vi "AMSServer.vi"() -> ()   [LabVIEW 2013]
uses:
  Controls/Enum - AMSServer State.ctl
  Controls/General Settings - AMS.ctl
  Controls/Configure Parameters - AMS.ctl
  Controls/Simulate Parameters - AMS.ctl
  Controls/DB - [AMS].[Execute].[Message] ColNames.ctl
  Controls/DB - OpenClose.ctl
  Controls/DB - [AMS].[Execute].[Message] Enum.ctl
  Controls/DB - AMS Execute EventLog.ctl
  Controls/DB - [AMS].[Execute].[EventLog] Enum.ctl
  <vilib>/Utility/miscctls.llb/LVPointTypeDef.ctl
  Controls/Global AMS.vi
panel:
  out "ini":errorcluster
  out "Application Directory":path=path "C:/Users/CK/workspace/LabVIEW/Stress Relief Temperature Recording"
  out "Application:Name":string="LabVIEW.exe"
  in  "Debug Close":bool caption="Close"
  out "EventLog":string
  in  "Simulate Parameters":T1={"Simulate Send SMS"=TRUE, "Simulate Stringx [Unicode]"=FALSE, "Simulate Send Email"=TRUE, "Simulate Email Fail"=FALSE, "Simulate SMS Fail"=FALSE}
  out "AMS Configure Parameters":T2
  out "AMS General Settings":T3
  out "AMS.Execute.Message":string[](array[string])
  out "Config.GeneralSetting":string[][](array[string])
  out "# elements in Q":i32
  out "# of elements DeQueued":i32
  out "Time has Elapsed":bool
  out "Q Error":errorcluster
  out "State Machine for AMSServer Main Process":T4
  out "Stop Flag":bool
  out "DeQ MessageNo":string
  out "SUMMARY":errorcluster
  out "Last MessageNo Checked":string
  in  "Time Target (s)":dbl=1.0
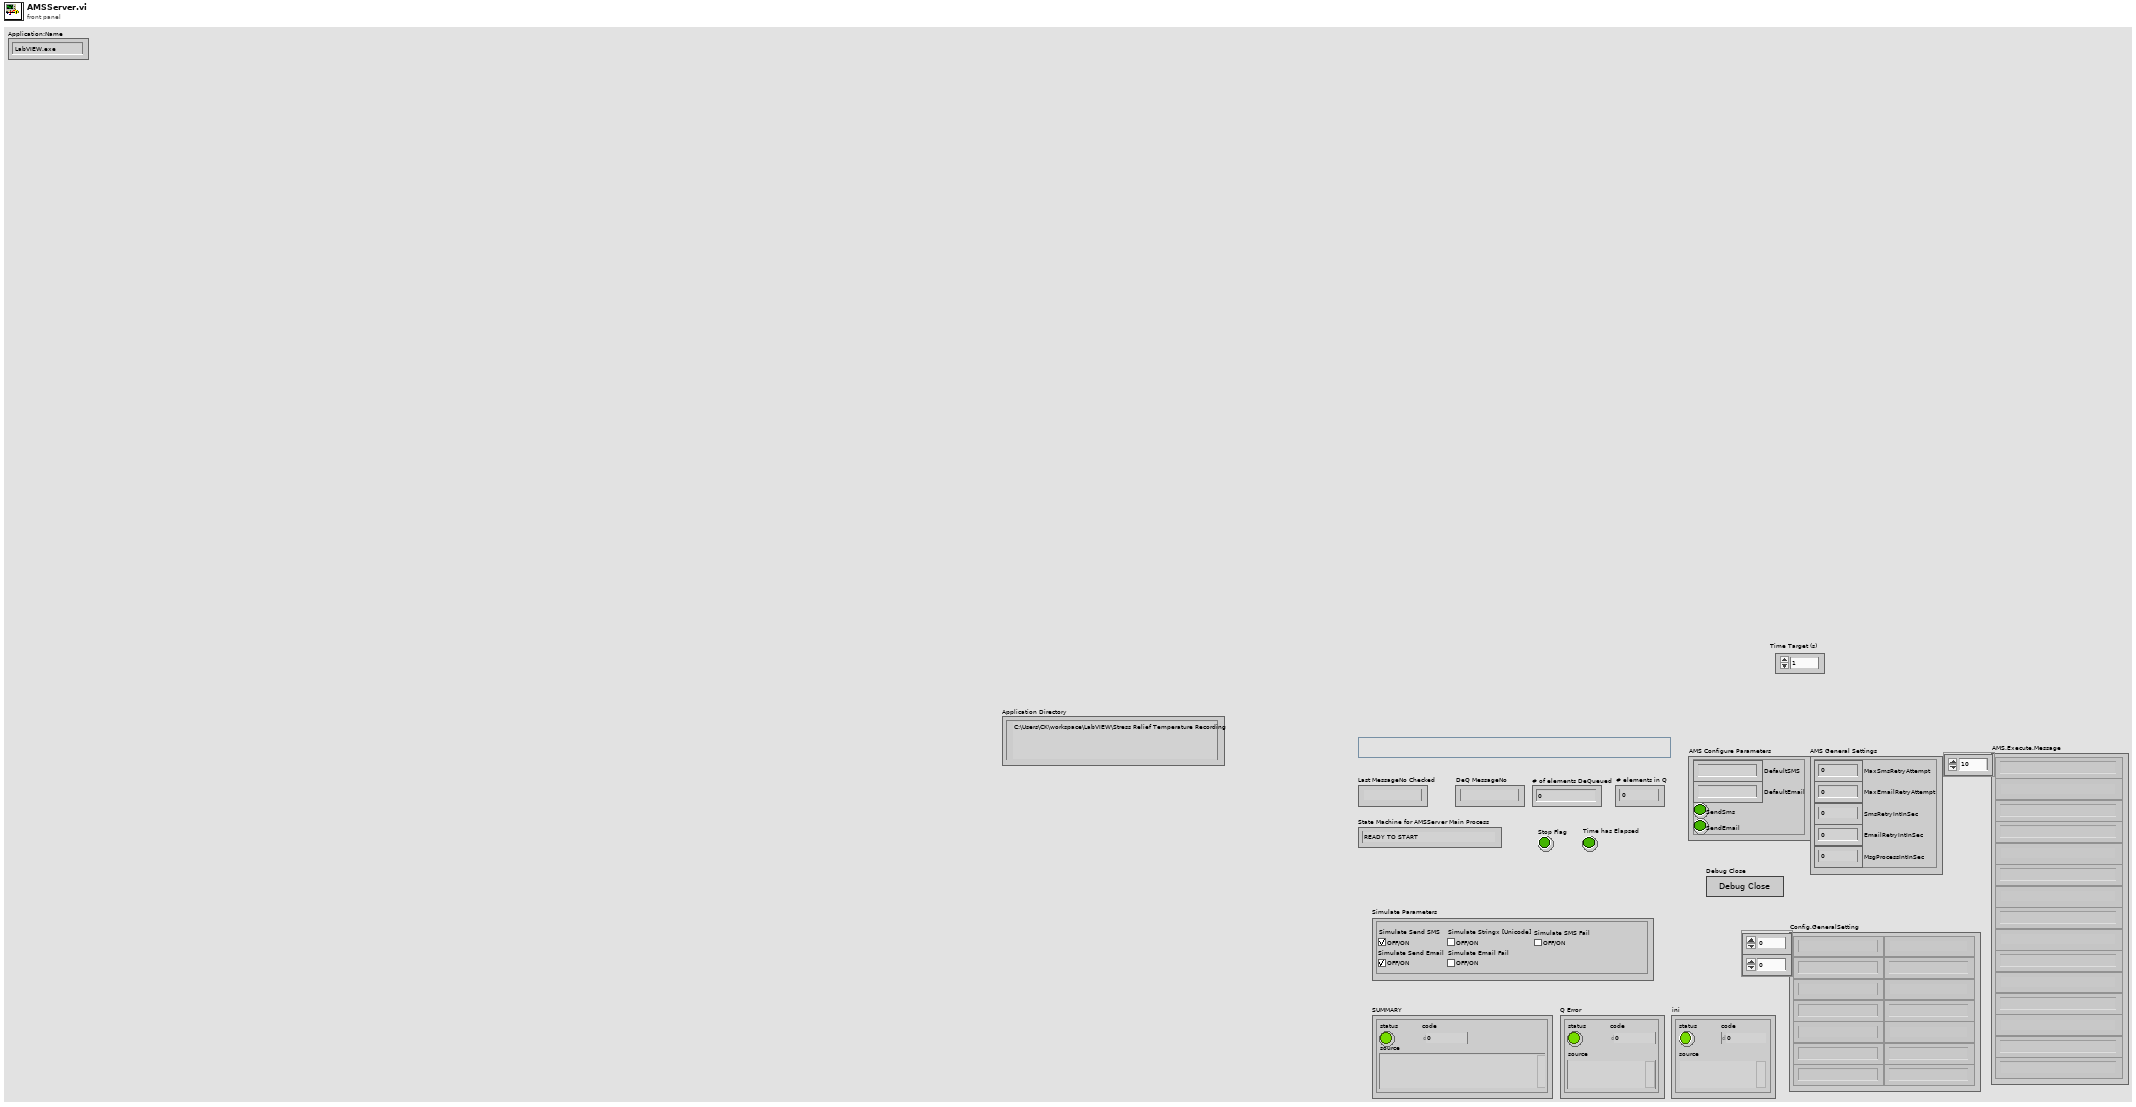
[diagram p1: front panel]
types:
  T1 = typedef "Simulate Parameters - AMS.ctl" = cluster{"Simulate Send SMS":bool, "Simulate Stringx [Unicode]":bool, "Simulate Send Email":bool, "Simulate Email Fail":bool, "Simulate SMS Fail":bool}
  T2 = typedef "Configure Parameters - AMS.ctl" = cluster{"DefaultSMS":string, "DefaultEmail":string, "SendSms":bool, "SendEmail":bool}
  T3 = typedef "General Settings - AMS.ctl" = cluster{"MaxSmsRetryAttempt":i32, "MaxEmailRetryAttempt":i32, "SmsRetryIntInSec":i32, "EmailRetryIntInSec":i32, "MsgProcessIntInSec":i32}
  T4 = typedef "Enum - AMSServer State.ctl" = enum16{"READY TO START", "RUNNING Process", "QUIT"}
  T5 = typedef "LVPointTypeDef.ctl" = cluster{"Horizontal":i16, "Vertical":i16}
  T6 = typedef "DB - AMS Execute EventLog.ctl" = cluster{"EventType":string, "Source":string, "UserId":string, "Computer":string, "CreatedOn":string, "Remarks1":string}
  T7 = typedef "DB - [AMS].[Execute].[EventLog] Enum.ctl" = enum16{"SELECT 'CreatedOn'", "SELECT 'LastMessageNo'", "INSERT"}
  T8 = typedef "Connection Information Cluster.ctl" = cluster{"Connection ":string, "Username":string, "Password":string}
  T9 = cluster{"Show LabVIEW Error":bool, "Simulate Send SMS":bool, "Simulate Send Email":bool, "Resizable":bool}
  T10 = typedef "DB - [AMS].[Execute].[Message] ColNames.ctl" = enum16{"[MessageNo]", "[LanguageId]", "[SoftwareSolutionId]", "[SoftwareSolutionName]", "[PlantId]", "[SystemId]", "[StationId]", "[MessageLogNo]", "[ReceivedOn]", "[MessageCode]", "[ShortDescription]", "[Message]", "[SmsMessage]", "[SuppMessage1]", "[SuppMessage2]", "[SuppMessage3]", "[TransactionNo]", "[TransactionRunNo]", "[MessageInitiator]", "[Remarks]", "[MsgCreatedOn]", "[IsToSendSms]", "[IsToSendEmail]", "[IsToSendCommMedium1]", "[IsToSendCommMedium2]", "[SmsContent]", "[EmailContent]", "[CommMed1Content]", "[CommMed2Content]", "[MobileNos]", "[EmailAddresses]", "[CommMedium1Ids]", "[CommMedium2Ids]", "[LastAttemptedCommMed]", "[LastAttemptedNo]", "[LastAttemptedOn]", "[IsSmsSent]", "[IsEmailSent]", "[IsCommMedium1Sent]", "[IsCommMedium2Sent]", "[OverallSentStatus]", "[StatusUpdatedOn]", "[IsArchived]"}
  T11 = typedef "DB - [AMS].[Execute].[Message] Enum.ctl" = enum16{"SELECT", "SELECT (Multi-Conditions)", "UPDATE", "RE-INSERT"}
  T12 = typedef "DB - OpenClose.ctl" = cluster{"Open":bool, "Close":bool}
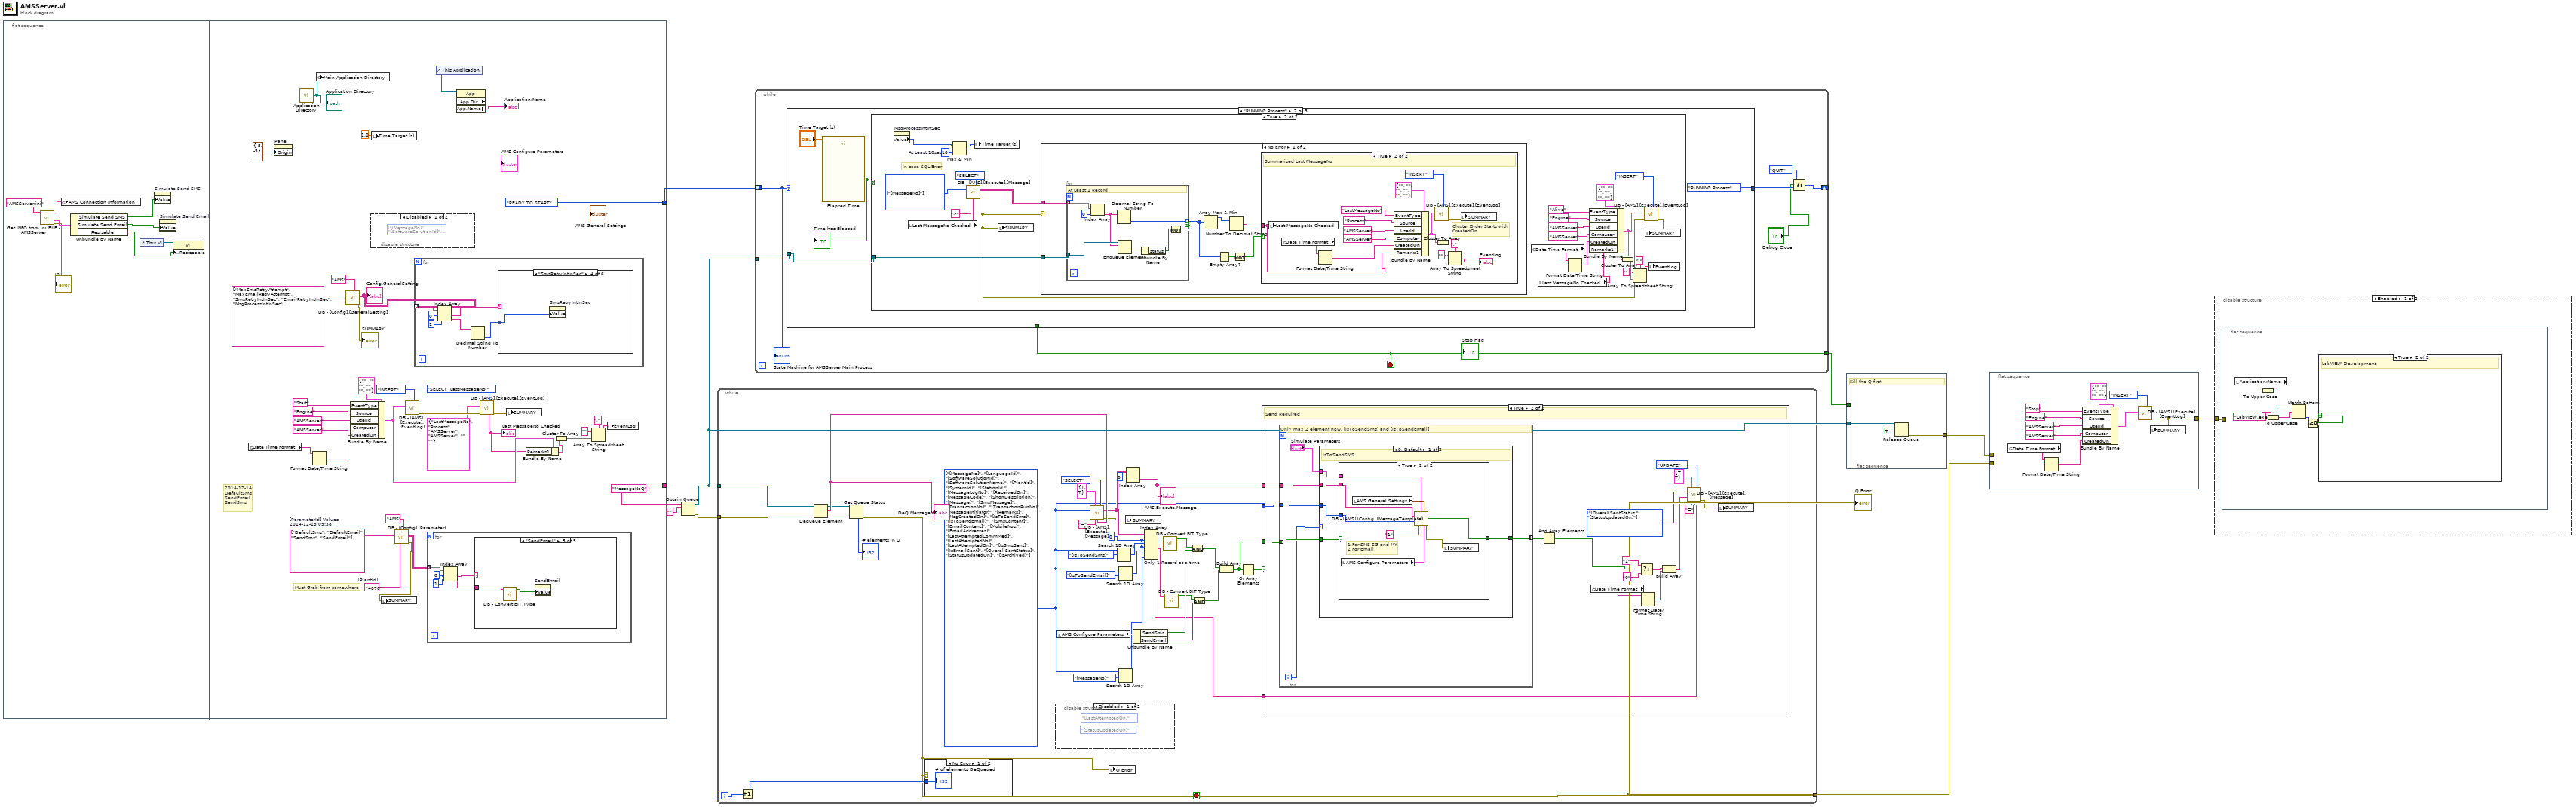
[diagram p0: block diagram]
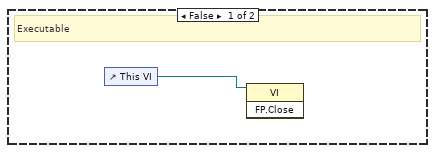
[diagram p2: hidden frame]
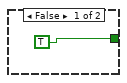
[diagram p6: hidden frame]
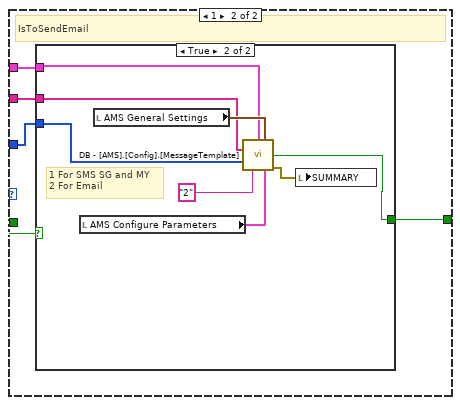
[diagram p7: hidden frame]
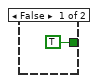
[diagram p8: hidden frame]
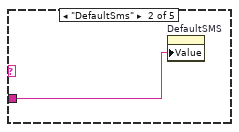
[diagram p11: hidden frame]
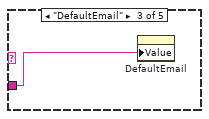
[diagram p12: hidden frame]
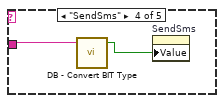
[diagram p13: hidden frame]
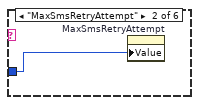
[diagram p15: hidden frame]
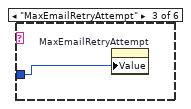
[diagram p16: hidden frame]
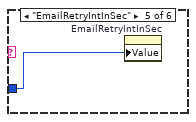
[diagram p17: hidden frame]
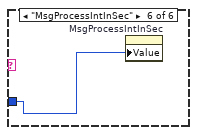
[diagram p18: hidden frame]
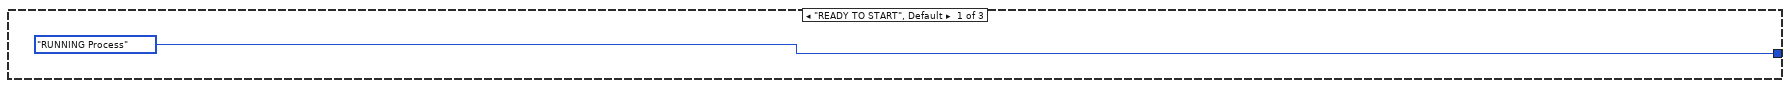
[diagram p20: hidden frame]
diagram:
  n1 = flat-sequence {
    tunnel: [Enum_-_AMSServer_State."READY TO START" ("State Machine for AMSServer Main Process")] -> w9
    tunnel: ["MessageNoQ" ("name (unnamed)")] -> w2
    frame #0 {
      n2 = call "Get INFO from ini FILE - AMSServer.vi"("ini Name"="AMSServer.ini") -> ("AMS Connection Information"=w16:T8, "Settings Boolean"=w17:T9, "Error Out"=→"ini":errorcluster)  [unwired: 9 in, 3 out]
      n3 = global write "Global AMS.vi" "AMS Connection Information"(w16) -> ()
      n4 = Unbundle By Name(w17) -> ("Simulate Send SMS"=w14:bool, "Simulate Send Email"=w13:bool, "Resizable"=w10:bool)
      n5 = control-ref of="This VI"() -> (w11:refnum<vi>)
      n6 = property on="Simulate Send SMS" class="Bool (strict)"("Value"=w14) -> ()  [unwired: 2 in, 2 out]
      n7 = property on="Simulate Send Email" class="Bool (strict)"("Value"=w13) -> ()  [unwired: 2 in, 2 out]
      n8 = property class="VI"(reference=w11, "Front Panel.Resizeable"=w10) -> ()  [unwired: 1 in, 2 out]
    }
    frame #1 {
      w38 = "4070"  # [PlantId]
      w40 = string[] ["DefaultSms", "DefaultEmail", "SendSms", "SendEmail"]  # [ParameterId] Values 2014-12-15 09:38
      # "2014-12-14\nDefaultSms\nSendEmail\nSendSms"
      # "Must Grab from somewhere"
      n9 = global read "Global AMS.vi" "Date Time Format"() -> (w43:string)
      n10 = property on="Pane" class="Pane"("Origin"=T5 {"Horizontal"=-5, "Vertical"=-5}) -> ()  [unwired: 2 in, 2 out]
      n11 = call <vilib>:"Application Directory.vi"() -> ("Application Directory"=w24:path)
      "Application Directory" <- w24
      n12 = Format Date/Time String(time format string (%c)=w43) -> (date/time string=w42:string)  [unwired: 2 in]
      n13 = global write "Global AMS.vi" "Main Application Directory"(w24) -> ()
      n14 = call "DB - [Config].[GeneralSetting].vi"("Application"="AMS", "[SettingId] Values"=string[] ["MaxSmsRetryAttempt", "MaxEmailRetryAttempt", "SmsRetryIntInSec", "EmailRetryIntInSec", "MsgProcessIntInSec"]) -> ("SUMMARY"=→"SUMMARY":errorcluster, "2D data"=w26:string[][])  [unwired: 7 in, 1 out]
      "Config.GeneralSetting" <- w26
      n15 = Bundle By Name(cluster=T6 {"EventType"="", "Source"="", "UserId"="", "Computer"="", "CreatedOn"="", "Remarks1"=""} ("AMS Execute EventLog"), "EventType"="Start", "Source"="Engine", "UserId"="AMSServer", "Computer"="AMSServer", "CreatedOn"=w42) -> (w21:T6)
      n16 = disable-structure shown="Disabled" {
        frame Disabled {
          (unwired) T10[] [enum."[MessageNo]", enum."[SoftwareSolutionId]", enum."[SoftwareSolutionName]", enum."[PlantId]", enum."[MessageLogNo]", enum."[ReceivedOn]", enum."[MessageCode]", enum."[ShortDescription]", enum."[Message]", enum."[SmsMessage]", enum."[TransactionNo]", enum."[TransactionRunNo]", enum."[MessageInitiator]", enum."[Remarks]", enum."[MsgCreatedOn]", enum."[IsToSendSms]", enum."[IsToSendEmail]", enum."[SmsContent]", enum."[EmailContent]", enum."[MobileNos]", enum."[EmailAddresses]"] items=["[MessageNo]", "[LanguageId]", "[SoftwareSolutionId]", "[SoftwareSolutionName]", "[PlantId]", "[SystemId]", "[StationId]", "[MessageLogNo]", "[ReceivedOn]", "[MessageCode]", "[ShortDescription]", "[Message]", "[SmsMessage]", "[SuppMessage1]", "[SuppMessage2]", "[SuppMessage3]", "[TransactionNo]", "[TransactionRunNo]", "[MessageInitiator]", "[Remarks]", "[MsgCreatedOn]", "[IsToSendSms]", "[IsToSendEmail]", "[IsToSendCommMedium1]", "[IsToSendCommMedium2]", "[SmsContent]", "[EmailContent]", "[CommMed1Content]", "[CommMed2Content]", "[MobileNos]", "[EmailAddresses]", "[CommMedium1Ids]", "[CommMedium2Ids]", "[LastAttemptedCommMed]", "[LastAttemptedNo]", "[LastAttemptedOn]", "[IsSmsSent]", "[IsEmailSent]", "[IsCommMedium1Sent]", "[IsCommMedium2Sent]", "[OverallSentStatus]", "[StatusUpdatedOn]", "[IsArchived]"] ("AMS Execute Message ColNames")
        }
        frame Enabled {
        }
      }
      n17 = local write "Time Target (s)"(1.0 ("Time Target (s)")) -> ()
      n18 = call "DB - [Config].[Parameter].vi"("Application"="AMS", "[PlantId]"=w38, "[ParameterId] Values"=w40) -> ("SUMMARY"=w18:errorcluster, "2D data"=w25:string[][])  [unwired: 6 in, 1 out]
      n19 = local write "SUMMARY"(w18) -> ()
      n20 = call "DB - [AMS].[Execute].[EventLog].vi"("DB - [AMS].[Execute].[EventLog]"=DB_-_[AMS].[Execute].[EventLog]_Enum."INSERT", "AMS Execute EventLog"=w21) -> ("SUMMARY"=w35:errorcluster)  [unwired: 5 in, 4 out]
      n21 = for {
        tunnel: w26 -> [w69] mode=indexing
        n22 = Index Array(array=w69, index #1=0 ("index"), index #2=1 ("index")) -> (element #1=w67:string, element #2=w65:string)
        n23 = Decimal String To Number(string=w65) -> (number=w64:i32)  [unwired: 2 in, 1 out]
        n24 = case shown="\"SmsRetryIntInSec\"" w67 {
          tunnel: w64 -> [_ w70 w71 w72 w73 w74]
          frame "False", Default {
          }
          frame "MaxSmsRetryAttempt" {
            n25 = property on="MaxSmsRetryAttempt" class="DigNum (strict)"("Value"=w70) -> ()  [unwired: 2 in, 2 out]
          }
          frame "MaxEmailRetryAttempt" {
            n26 = property on="MaxEmailRetryAttempt" class="DigNum (strict)"("Value"=w71) -> ()  [unwired: 2 in, 2 out]
          }
          frame "SmsRetryIntInSec" {
            n27 = property on="SmsRetryIntInSec" class="DigNum (strict)"("Value"=w72) -> ()  [unwired: 2 in, 2 out]
          }
          frame "EmailRetryIntInSec" {
            n28 = property on="EmailRetryIntInSec" class="DigNum (strict)"("Value"=w73) -> ()  [unwired: 2 in, 2 out]
          }
          frame "MsgProcessIntInSec" {
            n29 = property on="MsgProcessIntInSec" class="DigNum (strict)"("Value"=w74) -> ()  [unwired: 2 in, 2 out]
          }
        }
      }
      n30 = for {
        tunnel: w25 -> [w57] mode=indexing
        n31 = Index Array(array=w57, index #1=0 ("index"), index #2=1 ("index")) -> (element #1=w55:string, element #2=w53:string)
        n32 = case shown="\"SendEmail\"" w55 {
          tunnel: w53 -> [_ w58 w59 w61 w63]
          frame "", Default {
          }
          frame "DefaultSms" {
            n33 = property on="DefaultSMS" class="Str"("Value"=w58) -> ()  [unwired: 2 in, 2 out]
          }
          frame "DefaultEmail" {
            n34 = property on="DefaultEmail" class="Str"("Value"=w59) -> ()  [unwired: 2 in, 2 out]
          }
          frame "SendSms" {
            n35 = call "DB - Convert BIT Type.vi"("BIT Type (eg Inactive)"=w61) -> ("Boolean"=w60:bool)  [unwired: 2 in, 2 out]
            n36 = property on="SendSms" class="Bool (strict)"("Value"=w60) -> ()  [unwired: 2 in, 2 out]
          }
          frame "SendEmail" {
            n37 = call "DB - Convert BIT Type.vi"("BIT Type (eg Inactive)"=w63) -> ("Boolean"=w62:bool)  [unwired: 2 in, 2 out]
            n38 = property on="SendEmail" class="Bool (strict)"("Value"=w62) -> ()  [unwired: 2 in, 2 out]
          }
        }
      }
      n39 = control-ref of="This Application"() -> (w23:refnum<vi>)
      n40 = property class="App" props=["App.Dir", "App.Name"](reference=w23) -> ("App.Name"=→"Application:Name":string)  [unwired: 1 in, 3 out]
      n41 = call "DB - [AMS].[Execute].[EventLog].vi"("DB - [AMS].[Execute].[EventLog]"=DB_-_[AMS].[Execute].[EventLog]_Enum."SELECT 'LastMessageNo'", "error in (no error)"=w35, "AMS Execute EventLog"=T6 {"EventType"="LastMessageNo", "Source"="Process", "UserId"="AMSServer", "Computer"="AMSServer", "CreatedOn"="", "Remarks1"=""}) -> ("SUMMARY"=w34:errorcluster, "[LastMessageNo]"=w20:string)  [unwired: 4 in, 3 out]
      "Last MessageNo Checked" <- w20
      n42 = local write "SUMMARY"(w34) -> ()
      n43 = Bundle By Name(cluster=w21, "Remarks1"=w20) -> (w19:T6)
      n44 = Cluster To Array(cluster=w19) -> (array=w30:string[])
      n45 = Array To Spreadsheet String(delimiter (Tab)=",", array=w30, 3:"" ("format string")) -> (spreadsheet string=w32:string)
      n46 = local write "EventLog"(w32) -> ()
    }
  }
  n47 = Obtain Queue(name (unnamed)=w2, element data type="") -> (queue out=w6:refnum<queue>, error out=w8:errorcluster)  [unwired: 3 in, 1 out]
  n48 = while {
    tunnel: w6 -> [w104]
    tunnel: w8 -> [w110]
    tunnel: [w96] -> w3
    i -> [w107]
    stop <- w96 stop-if-true
    w78 = 0 ("index (row)")
    w75 = T10[] [enum."[MessageNo]", enum."[LanguageId]", enum."[SoftwareSolutionId]", enum."[SoftwareSolutionName]", enum."[PlantId]", enum."[SystemId]", enum."[StationId]", enum."[MessageLogNo]", enum."[ReceivedOn]", enum."[MessageCode]", enum."[ShortDescription]", enum."[Message]", enum."[SmsMessage]", enum."[TransactionNo]", enum."[TransactionRunNo]", enum."[MessageInitiator]", enum."[Remarks]", enum."[MsgCreatedOn]", enum."[IsToSendSms]", enum."[IsToSendEmail]", enum."[SmsContent]", enum."[EmailContent]", enum."[MobileNos]", enum."[EmailAddresses]", enum."[LastAttemptedCommMed]", enum."[LastAttemptedNo]", enum."[LastAttemptedOn]", enum."[IsSmsSent]", enum."[IsEmailSent]", enum."[OverallSentStatus]", enum."[StatusUpdatedOn]", enum."[IsArchived]"] items=["[MessageNo]", "[LanguageId]", "[SoftwareSolutionId]", "[SoftwareSolutionName]", "[PlantId]", "[SystemId]", "[StationId]", "[MessageLogNo]", "[ReceivedOn]", "[MessageCode]", "[ShortDescription]", "[Message]", "[SmsMessage]", "[SuppMessage1]", "[SuppMessage2]", "[SuppMessage3]", "[TransactionNo]", "[TransactionRunNo]", "[MessageInitiator]", "[Remarks]", "[MsgCreatedOn]", "[IsToSendSms]", "[IsToSendEmail]", "[IsToSendCommMedium1]", "[IsToSendCommMedium2]", "[SmsContent]", "[EmailContent]", "[CommMed1Content]", "[CommMed2Content]", "[MobileNos]", "[EmailAddresses]", "[CommMedium1Ids]", "[CommMedium2Ids]", "[LastAttemptedCommMed]", "[LastAttemptedNo]", "[LastAttemptedOn]", "[IsSmsSent]", "[IsEmailSent]", "[IsCommMedium1Sent]", "[IsCommMedium2Sent]", "[OverallSentStatus]", "[StatusUpdatedOn]", "[IsArchived]"] ("AMS Execute Message ColNames")
    n49 = Increment(x=w107) -> (x+1=w106:i32)
    n50 = Dequeue Element(queue=w104, error in (no error)=w110) -> (queue out=w103:refnum<queue>, element=w108:string, error out=w102:errorcluster)  [unwired: 1 in, 1 out]
    "DeQ MessageNo" <- w108
    n51 = Get Queue Status(queue=w103, error in (no error)=w102) -> (error out=w96:errorcluster, # elements in queue=→"# elements in Q":i32)  [unwired: 1 in, 6 out]
    n52 = case shown="No Error" w96 {
      tunnel: w106 -> [w162 _]
      frame No Error {
        "# of elements DeQueued" <- w162
      }
      frame Error {
      }
    }
    n53 = disable-structure shown="Disabled" {
      frame Disabled {
        (unwired) DB_-_[AMS].[Execute].[Message]_ColNames."[StatusUpdatedOn]" ("[AMS].[Execute].[Message] ColNames")
        (unwired) DB_-_[AMS].[Execute].[Message]_ColNames."[LastAttemptedOn]" ("[AMS].[Execute].[Message] ColNames")
      }
      frame Enabled {
      }
    }
    n54 = local read "AMS Configure Parameters"() -> (w86:T2)
    n55 = call "DB - [AMS].[Execute].[Message].vi"("DB Connection"=T12 {"Open"=TRUE, "Close"=TRUE}, "DB - [AMS].[Execute].[Message] Enum"=DB_-_[AMS].[Execute].[Message]_Enum."SELECT", "AMS Execute Message ColNames"=w75, "<SIGN>"="=", "[MessageNo]"=w108) -> ("2D data"=w94:string[][], "SUMMARY"=w87:errorcluster)  [unwired: 7 in, 2 out]
    n56 = local write "Q Error"(w96) -> ()
    n57 = Search 1D Array(1D array=w75, element=DB_-_[AMS].[Execute].[Message]_ColNames."[IsToSendSms]") -> (index of element=w99:i32)  [unwired: 1 in]
    n58 = Search 1D Array(1D array=w75, element=DB_-_[AMS].[Execute].[Message]_ColNames."[IsToSendEmail]") -> (index of element=w98:i32)  [unwired: 1 in]
    n59 = Search 1D Array(1D array=w75, element=DB_-_[AMS].[Execute].[Message]_ColNames."[MessageNo]") -> (index of element=w77:i32)  [unwired: 1 in]
    n60 = local write "SUMMARY"(w87) -> ()
    n61 = Index Array(array=w94, index (row)=0) -> (element=w90:string[])  [unwired: 1 in]
    "AMS.Execute.Message" <- w90
    n62 = Unbundle By Name(w86) -> ("SendSms"=w84:bool, "SendEmail"=w81:bool)
    n63 = Index Array "Only 1 Record at a time"(array=w94, index (row) #1=w78, index (col) #1=w99, index (row) #2=w78, index (col) #2=w98, index (row) #3=w78, index (col) #3=w77) -> (element #1=w97:string, element #2=w105:string, element #3=w76:string)
    n64 = call "DB - Convert BIT Type.vi"("BIT Type (eg Inactive)"=w97) -> ("Boolean"=w85:bool)  [unwired: 2 in, 2 out]
    n65 = call "DB - Convert BIT Type.vi"("BIT Type (eg Inactive)"=w105) -> ("Boolean"=w82:bool)  [unwired: 2 in, 2 out]
    n66 = And(x=w85, y=w84) -> (x .and. y?=w83:bool)
    n67 = And(x=w82, y=w81) -> (x .and. y?=w80:bool)
    n68 = Build Array(w83, w80) -> (w91:bool[])
    n69 = Or Array Elements(Boolean array=w91) -> (logical OR=w92:bool)
    n70 = case shown="True" w92 {
      tunnel: w75 -> [_ w127]
      tunnel: w91 -> [_ w126]
      tunnel: w90 -> [_ w125]
      tunnel: w76 -> [_ w119]
      frame False {
      }
      frame True {
        w121 = T10[] [enum."[OverallSentStatus]", enum."[StatusUpdatedOn]"] items=["[MessageNo]", "[LanguageId]", "[SoftwareSolutionId]", "[SoftwareSolutionName]", "[PlantId]", "[SystemId]", "[StationId]", "[MessageLogNo]", "[ReceivedOn]", "[MessageCode]", "[ShortDescription]", "[Message]", "[SmsMessage]", "[SuppMessage1]", "[SuppMessage2]", "[SuppMessage3]", "[TransactionNo]", "[TransactionRunNo]", "[MessageInitiator]", "[Remarks]", "[MsgCreatedOn]", "[IsToSendSms]", "[IsToSendEmail]", "[IsToSendCommMedium1]", "[IsToSendCommMedium2]", "[SmsContent]", "[EmailContent]", "[CommMed1Content]", "[CommMed2Content]", "[MobileNos]", "[EmailAddresses]", "[CommMedium1Ids]", "[CommMedium2Ids]", "[LastAttemptedCommMed]", "[LastAttemptedNo]", "[LastAttemptedOn]", "[IsSmsSent]", "[IsEmailSent]", "[IsCommMedium1Sent]", "[IsCommMedium2Sent]", "[OverallSentStatus]", "[StatusUpdatedOn]", "[IsArchived]"] ("AMS Execute Message ColNames")
        # "Send Required"
        n71 = for {
          tunnel: w127 -> [w133]
          tunnel: w126 -> [w132] mode=indexing
          tunnel: w125 -> [w130]
          tunnel: [w128] -> w124 mode=indexing
          i -> [w131]
          # "Only max 2 element now. [IsToSendSms] and [IsToSendEmail]"
          n72 = case shown="0, Default" w131 {
            tunnel: w133 -> [w137 w151]
            tunnel: w132 -> [w138 w152]
            tunnel: w130 -> [w136 w150]
            tunnel: "Simulate Parameters" -> [w135 w149]
            tunnel: [w134 w148] -> w128
            frame 0, Default {
              # "IsToSendSMS"
              n73 = case shown="True" w138 {
                tunnel: w137 -> [_ w147]
                tunnel: w136 -> [_ w146]
                tunnel: w135 -> [_ w141]
                tunnel: [TRUE w140] -> w134
                frame False {
                }
                frame True {
                  # "1 For SMS SG and MY\n2 For Email"
                  n74 = local read "AMS Configure Parameters"() -> (w144:T2)
                  n75 = local read "AMS General Settings"() -> (w143:T3)
                  n76 = call "DB - [AMS].[Config].[MessageTemplate].vi"("Simulate Parameters"=w141, "AMS General Settings"=w143, "AMS.Execute.Message"=w146, "AMS Execute Message ColNames"=w147, "[CommMediumId]"="1", "AMS Configure Parameters"=w144) -> ("All SMS/Email Delivered OK"=w140:bool, "SUMMARY"=w142:errorcluster)  [unwired: 6 in, 2 out]
                  n77 = local write "SUMMARY"(w142) -> ()
                }
              }
            }
            frame 1 {
              # "IsToSendEmail"
              n78 = case shown="True" w152 {
                tunnel: w151 -> [_ w160]
                tunnel: w150 -> [_ w156]
                tunnel: w149 -> [_ w155]
                tunnel: [TRUE ("All SMS/Email Delivered OK") w154] -> w148
                frame False {
                }
                frame True {
                  # "1 For SMS SG and MY\n2 For Email"
                  n79 = local read "AMS Configure Parameters"() -> (w158:T2)
                  n80 = local read "AMS General Settings"() -> (w159:T3)
                  n81 = call "DB - [AMS].[Config].[MessageTemplate].vi"("Simulate Parameters"=w155, "AMS General Settings"=w159, "AMS.Execute.Message"=w156, "AMS Execute Message ColNames"=w160, "[CommMediumId]"="2", "AMS Configure Parameters"=w158) -> ("All SMS/Email Delivered OK"=w154:bool, "SUMMARY"=w157:errorcluster)  [unwired: 6 in, 2 out]
                  n82 = local write "SUMMARY"(w157) -> ()
                }
              }
            }
          }
        }
        n83 = And Array Elements(Boolean array=w124) -> (logical AND=w113:bool)
        n84 = global read "Global AMS.vi" "Date Time Format"() -> (w118:string)
        n85 = Select(t="1", s=w113, f="0") -> (s? t:f=w115:string)
        n86 = Format Date/Time String(time format string (%c)=w118) -> (date/time string=w114:string)  [unwired: 2 in]
        n87 = Build Array(w115, w114) -> (w112:string[])
        n88 = call "DB - [AMS].[Execute].[Message].vi"("DB Connection"=T12 {"Open"=TRUE, "Close"=TRUE}, "DB - [AMS].[Execute].[Message] Enum"=DB_-_[AMS].[Execute].[Message]_Enum."UPDATE", "AMS Execute Message ColNames"=w121, "<Data> (0xFFFE autodetect)"=w112, "<SIGN>"="=", "[MessageNo]"=w119) -> ("SUMMARY"=w111:errorcluster)  [unwired: 6 in, 3 out]
        n89 = local write "SUMMARY"(w111) -> ()
      }
    }
  }
  "Q Error" <- w3
  n90 = while {
    shift-right: [w165] -> _
    shift-left: w9 -> [w169]
    tunnel: w6 -> [w168]
    tunnel: [w164] -> w5
    stop <- w164 stop-if-true
    n91 = case shown="\"RUNNING Process\"" w169 {
      tunnel: [Enum_-_AMSServer_State."RUNNING Process" ("State Machine for AMSServer Main Process") Enum_-_AMSServer_State."RUNNING Process" ("State Machine for AMSServer Main Process") _] -> w166
      tunnel: [_ _ TRUE] -> w164
      tunnel: w168 -> [_ w172 _]
      frame "READY TO START", Default {
      }
      frame "RUNNING Process" {
        n92 = call "Elapsed Time"("Time Target (s)"="Time Target (s)") -> ("Time has Elapsed"=w173:bool)  [unwired: 11 in, 7 out]
        "Time has Elapsed" <- w173
        n93 = case shown="True" w173 {
          tunnel: w172 -> [_ w197]
          frame False {
          }
          frame True {
            w183 = 10  # At Least 10sec
            w199 = T10[] [enum."[MessageNo]"] items=["[MessageNo]", "[LanguageId]", "[SoftwareSolutionId]", "[SoftwareSolutionName]", "[PlantId]", "[SystemId]", "[StationId]", "[MessageLogNo]", "[ReceivedOn]", "[MessageCode]", "[ShortDescription]", "[Message]", "[SmsMessage]", "[SuppMessage1]", "[SuppMessage2]", "[SuppMessage3]", "[TransactionNo]", "[TransactionRunNo]", "[MessageInitiator]", "[Remarks]", "[MsgCreatedOn]", "[IsToSendSms]", "[IsToSendEmail]", "[IsToSendCommMedium1]", "[IsToSendCommMedium2]", "[SmsContent]", "[EmailContent]", "[CommMed1Content]", "[CommMed2Content]", "[MobileNos]", "[EmailAddresses]", "[CommMedium1Ids]", "[CommMedium2Ids]", "[LastAttemptedCommMed]", "[LastAttemptedNo]", "[LastAttemptedOn]", "[IsSmsSent]", "[IsEmailSent]", "[IsCommMedium1Sent]", "[IsCommMedium2Sent]", "[OverallSentStatus]", "[StatusUpdatedOn]", "[IsArchived]"] ("AMS Execute Message ColNames")
            # "In case SQL Error"
            n94 = property on="MsgProcessIntInSec" class="DigNum (strict)"() -> ("Value"=w176:i32)  [unwired: 2 in, 2 out]
            n95 = local read "Last MessageNo Checked"() -> (w195:string)
            n96 = Max & Min(x=w176, y=w183) -> (max(x,y)=w182:i32)  [unwired: 1 out]
            n97 = call "DB - [AMS].[Execute].[Message].vi"("DB - [AMS].[Execute].[Message] Enum"=DB_-_[AMS].[Execute].[Message]_Enum."SELECT", "AMS Execute Message ColNames"=w199, "<SIGN>"=">", "[MessageNo]"=w195) -> ("2D data"=w198:string[][], "SUMMARY"=w185:errorcluster)  [unwired: 8 in, 2 out]
            n98 = local write "Time Target (s)"(w182) -> ()
            n99 = local write "SUMMARY"(w185) -> ()
            n100 = case shown="No Error" w185 {
              tunnel: w198 -> [w206 _]
              tunnel: w197 -> [w205 _]
              frame No Error {
                n101 = for {
                  tunnel: w206 -> [w229] mode=indexing
                  tunnel: w205 -> [w227]
                  tunnel: [w225] -> w202 mode=indexing if=w223
                  # "At Least 1 Record"
                  n102 = Index Array(array=w229, index=0) -> (element=w226:string)
                  n103 = Decimal String To Number(string=w226) -> (number=w225:i32)  [unwired: 2 in, 1 out]
                  n104 = Enqueue Element(queue=w227, element=w226) -> (error out=w224:errorcluster)  [unwired: 2 in, 2 out]
                  n105 = Unbundle By Name(w224) -> ("status"=w222:bool)
                  n106 = Not(x=w222) -> (.not. x?=w223:bool)
                }
                n107 = Array Max & Min(array=w202) -> (max value=w204:i32)  [unwired: 3 out]
                n108 = Empty Array?(array=w202) -> (empty?=w201:bool)
                n109 = Number To Decimal String(number=w204) -> (decimal integer string=w203:string)  [unwired: 1 in]
                n110 = Not(x=w201) -> (.not. x?=w200:bool)
                n111 = case shown="True" w200 {
                  tunnel: w203 -> [_ w214]
                  frame False {
                    # "Empty Array"
                  }
                  frame True {
                    # "Cluster Order Starts with\nCreatedOn"
                    # "Summarised Last MessageNo"
                    n112 = local write "Last MessageNo Checked"(w214) -> ()
                    n113 = global read "Global AMS.vi" "Date Time Format"() -> (w218:string)
                    n114 = Format Date/Time String(time format string (%c)=w218) -> (date/time string=w217:string)  [unwired: 2 in]
                    n115 = Bundle By Name(cluster=T6 {"EventType"="", "Source"="", "UserId"="", "Computer"="", "CreatedOn"="", "Remarks1"=""} ("AMS Execute EventLog"), "EventType"="LastMessageNo" ("Source"), "Source"="Process", "UserId"="AMSServer", "Computer"="AMSServer" ("UserId"), "CreatedOn"=w217, "Remarks1"=w214) -> (w211:T6)
                    n116 = call "DB - [AMS].[Execute].[EventLog].vi"("DB - [AMS].[Execute].[EventLog]"=DB_-_[AMS].[Execute].[EventLog]_Enum."INSERT", "AMS Execute EventLog"=w211) -> ("SUMMARY"=w221:errorcluster)  [unwired: 5 in, 4 out]
                    n117 = Cluster To Array(cluster=w211) -> (array=w210:string[])
                    n118 = Array To Spreadsheet String(delimiter (Tab)=",", array=w210, 3:"" ("format string")) -> (spreadsheet string=→"EventLog":string)
                    n119 = local write "SUMMARY"(w221) -> ()
                  }
                }
              }
              frame Error {
              }
            }
            n120 = global read "Global AMS.vi" "Date Time Format"() -> (w193:string)
            n121 = local read "Last MessageNo Checked"() -> (w175:string)
            n122 = Format Date/Time String(time format string (%c)=w193) -> (date/time string=w186:string)  [unwired: 2 in]
            n123 = Bundle By Name(cluster=T6 {"EventType"="", "Source"="", "UserId"="", "Computer"="", "CreatedOn"="", "Remarks1"=""} ("AMS Execute EventLog"), "EventType"="Alive", "Source"="Engine", "UserId"="AMSServer", "Computer"="AMSServer", "CreatedOn"=w186, "Remarks1"=w175) -> (w179:T6)
            n124 = Cluster To Array(cluster=w179) -> (array=w180:string[])
            n125 = Array To Spreadsheet String(delimiter (Tab)=",", array=w180, 3:"" ("format string")) -> (spreadsheet string=w177:string)
            n126 = call "DB - [AMS].[Execute].[EventLog].vi"("DB - [AMS].[Execute].[EventLog]"=DB_-_[AMS].[Execute].[EventLog]_Enum."INSERT", "error in (no error)"=w185, "AMS Execute EventLog"=w179) -> ("SUMMARY"=w184:errorcluster)  [unwired: 4 in, 4 out]
            n127 = local write "SUMMARY"(w184) -> ()
            n128 = local write "EventLog"(w177) -> ()
          }
        }
      }
      frame "QUIT" {
      }
    }
    "Stop Flag" <- w164
    n129 = Select(t=Enum_-_AMSServer_State."QUIT" ("State Machine for AMSServer Main Process"), s="Debug Close", f=w166) -> (s? t:f=w165:T4)
    "State Machine for AMSServer Main Process" <- w169
  }
  n130 = flat-sequence {
    tunnel: w6 -> [w233]
    tunnel: w5 -> [_]
    tunnel: [w231] -> w4
    frame #0 {
      # "Kill the Q first"
      n131 = Release Queue(queue=w233, force destroy? (F)=TRUE) -> (error out=w231:errorcluster)  [unwired: 1 in, 2 out]
    }
  }
  n132 = flat-sequence {
    tunnel: w4 -> [_]
    tunnel: w3 -> [_]
    tunnel: [w234] -> w1
    frame #0 {
      n133 = global read "Global AMS.vi" "Date Time Format"() -> (w237:string)
      n134 = Format Date/Time String(time format string (%c)=w237) -> (date/time string=w236:string)  [unwired: 2 in]
      n135 = Bundle By Name(cluster=T6 {"EventType"="", "Source"="", "UserId"="", "Computer"="", "CreatedOn"="", "Remarks1"=""} ("AMS Execute EventLog"), "EventType"="Stop", "Source"="Engine", "UserId"="AMSServer", "Computer"="AMSServer", "CreatedOn"=w236) -> (w242:T6)
      n136 = call "DB - [AMS].[Execute].[EventLog].vi"("DB - [AMS].[Execute].[EventLog]"=DB_-_[AMS].[Execute].[EventLog]_Enum."INSERT", "AMS Execute EventLog"=w242) -> ("SUMMARY"=w234:errorcluster)  [unwired: 5 in, 4 out]
      n137 = local write "SUMMARY"(w234) -> ()
    }
  }
  n138 = disable-structure shown="Enabled" {
    disable-tunnel: w1 -> [w244 _]
    frame Enabled {
      n139 = flat-sequence {
        tunnel: w244 -> [_]
        frame #0 {
          n140 = local read "Application:Name"() -> (w250:string)
          n141 = To Upper Case(1:w250) -> (0:w249:string)
          n142 = To Upper Case(1:"LabVIEW.exe" ("regular expression")) -> (0:w247:string)
          n143 = Match Pattern(string=w249, regular expression=w247) -> (offset past match=w246:i32)  [unwired: 1 in, 3 out]
          n144 = Greater Or Equal To 0?(x=w246) -> (x >= 0?=w245:bool)
          n145 = case shown="True" w245 {
            frame False {
              # "Executable"
              n146 = control-ref of="This VI"() -> (w251:refnum<vi>)
              n147 = invoke class="VI" method="FP.Close"(reference=w251) -> ()  [unwired: 2 in, 3 out]
            }
            frame True {
              # "LabVIEW Development"
            }
          }
        }
      }
    }
    frame Disabled {
    }
  }
